vi "AOM.vi"(1 "In":variant, 2 "Mode":u32(ring) items=["Open", "Close", "Begin", "End", "Get", "Set"]) -> (0 "Out":variant)   [LabVIEW 2014]
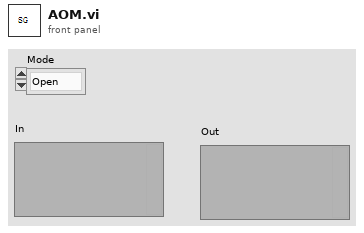
[diagram p1: front panel]
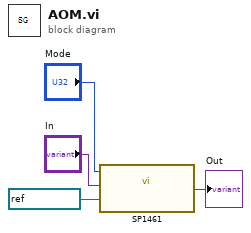
[diagram p0: block diagram]
diagram:
  n1 = call "SP1461.vi"("Port"=refnum<visa-resource-name> "COM13", "In"="In", "Mode"="Mode") -> ("Out"=→"Out":variant)
